vi "Multirecord Acquisition FPGA_20221228a.vi"() -> ()   [LabVIEW 2021]
doc: "Use this VI as a template for the reconfigurable oscilloscope acquisition design. The block diagram is divided into three main loops.\n\nRegister Bus: This loop initializes the registers that are needed to support the configuration of the device. The FIFO bus, on the left, allows all the other design libraries to communicate with one another. This loop is very important to support the proper behavior of the instrument design library components.\n\nAcquisition: Acquires data from the I/O channels and writes the data into the record memory using the <B>Write</B> VI of the Multirecord Acquisition instrument design library. This VI also evaluates the various acquisition triggers and decides whether to acquire each data value in record memory. The host level VI (Fetch Record.vi) can read acquired records from the DRAM. The data is stored in 2 DRAM banks, each with 768 MB of storage.\n\nFetch: The recorded data is retrieved when the <B>Fetch Single Record</B> VI is run from the host VI. The <B>Write to Fetch DMA FIFO</B> VI writes data to the acq.fetch fifo 0 to transmit record data form the FPGA to the record fetch VIs on the host. This DMA FIFO must have a predefined name based on the instance parameter. By default, it is 0 (since the associated terminal on the <B>Create Resources DRAM Write Read</B> VI is unwired), so the connected FIFO is named acq.fetch fifo 0."
uses:
  FPGA Interface Typedefinitions/Trigger Combination Type.ctl
  Host/Clusts/AllWindowsClust.ctl
  Host/Clusts/ChannelWindowClust.ctl
  Controls/Clust/WindowTriggerClust.ctl
  <instrlib>/_niInstr/Data Trigger/v1/Shared/Public/Level Configuration FXP(+-,18,1).ctl
  <instrlib>/_niInstr/Data Trigger/v1/Shared/Public/Level Configuration Trigger When.ctl
  <vilib>/Platform/TimedLoop/XDataNode/timing_clust.ctl
  <vilib>/Platform/TimedLoop/XDataNode/nitl_modes.ctl
  <vilib>/Platform/TimedLoop/XDataNode/wakeup.ctl
  Controls/Clust/All_acquisition_Resources.ctl
  <instrlib>/_niInstr/Multirecord Acquisition/Common/v1/FPGA/niInstr Multirecord Acquisition Common v1 FPGA.lvclass
  C:/Program Files (x86)/National Instruments/LabVIEW 2021/instr.lib/_niInstr/Multirecord Acquisition/Interface/v1/FPGA/niInstr Multirecord Acquisition v1 FPGA.lvclass
  Controls/Clust/Status_Booleans_Clust.ctl
  Controls/Clust/Trig_Config_Clust.ctl
  <instrlib>/_niInstr/FIFO Register Bus/v1/FPGA/niInstr FIFO Register Bus v1 FPGA.lvclass
  C:/Program Files (x86)/National Instruments/LabVIEW 2021/instr.lib/_niInstr/Instruction Framework/v1/FPGA/Interfaces/Instruction Producer/Instruction Producer.lvclass
  <vilib>/rvi/Emulation/niFpgaSctlEmulationGetInTimedLoop.vi
  <vilib>/rvi/Emulation/niFpgaEmulationReportErrorSimple.vi
  <vilib>/rvi/Emulation/niFpgaGetClockAttributes.vi
  <vilib>/rvi/Emulation/niFpgaCriticalErrorInLSC.vi
  <instrlib>/_niInstr/Multirecord Acquisition/Common/v1/FPGA/Private/Create Fetch DMA FIFO Resources U8x32.vi
  <instrlib>/_niInstr/Multirecord Acquisition/Common/v1/FPGA/Private/Create Resources DRAM U384x2 U768 Write Read.vi
  <instrlib>/_niInstr/Multirecord Acquisition/Interface/v1/FPGA/Private/Retrieve Record U16 Wrapper.vi
  <instrlib>/_niInstr/Multirecord Acquisition/Interface/v1/FPGA/Private/Write to Fetch DMA FIFO U16 Wrapper.vi
  <vilib>/rvi/eio/common/nirviEmuTemplateMethod_errors.vi
  <instrlib>/HSAI-RIO/Config/Group A/v1/FPGA/Digital Correction/Validate 8 Channel Data.vi
  <instrlib>/HSAI-RIO/Config/Group A/v1/FPGA/Digital Correction/Digital Correction (8 Ch).vi
  <instrlib>/HSAI-RIO/Config/Group A/v1/FPGA/Digital Correction/FIR Filter (8 Ch).vi
  DSP/SubVIs/Integer decimationx8ch.vi
  <vilib>/Platform/TimedLoop/XDataNode/XDataNode.xnode
  <vilib>/eio/EIONode/EIONode.xnode
  <instrlib>/_niInstr/Instruction Framework/v1/FPGA/Top Level Bus/Register Configuration/Register Configuration.lvclass
  <vilib>/Platform/TimedLoop/XDataNode/XDNodeRunTimeDep.lvlib
  <instrlib>/_niInstr/Multirecord Acquisition/Interface/v1/FPGA/niInstr Multirecord Acquisition v1 FPGA.lvclass
  <instrlib>/_niInstr/Basic Elements/v1/FPGA/niInstr Basic Elements v1 FPGA.lvlib
  <instrlib>/HSAI-RIO/Config/Group A/v1/FPGA/Digital Correction/Digital Correction.lvclass
  <instrlib>/HSAI-RIO/Config/Group A/v1/FPGA/Config Registers/Config Registers.lvclass
  FPGA Interface Typedefinitions/FPGA Interface Typedefinitions.lvlib
  C:/Program Files (x86)/National Instruments/LabVIEW 2021/instr.lib/_niInstr/Multirecord Acquisition/Common/v1/FPGA/niInstr Multirecord Acquisition Common v1 FPGA.lvclass
  Emulation/SubVIs/2 Element Generate Sine Cos Data FXP(+,-,14,1).vi
  <instrlib>/_niInstr/Data Trigger/v1/Shared/niInstr Data Trigger v1 Shared.lvlib
panel:
  in  "channel.enable mask":u16=65535 format="%.0b"
  in  "channel.number of channels":u8=8
  out "overflow 2":bool
  out "TrigCount 2":u32
  out "Trigger Index 2":u16
  out "TrigCfg 1":T1
  out "Trigger Index":u16
  out "TrigCount":u32
  out "TrigCfg 0":T1
  in  "ResetTrig":bool
  in  "UserTrig":T4
  in  "trigger.rearm delay":u16=2
  in  "start trigger":bool=TRUE
  in  "reset":bool
  in  "trigger.combination type":T6
  out "fifo reg bus data 0":u64
  out "fifo reg bus status 0":u32
  in  "fifo reg bus ctrl 0":u32
  out "overflow":bool
  in  "dsp.decimation factor":u16
  out "overload":bool
  # "Register Bus Controls"
  # "FPGA"
  # "DSP"
  # "Trigger"
  # "Unused controls included to make API work"
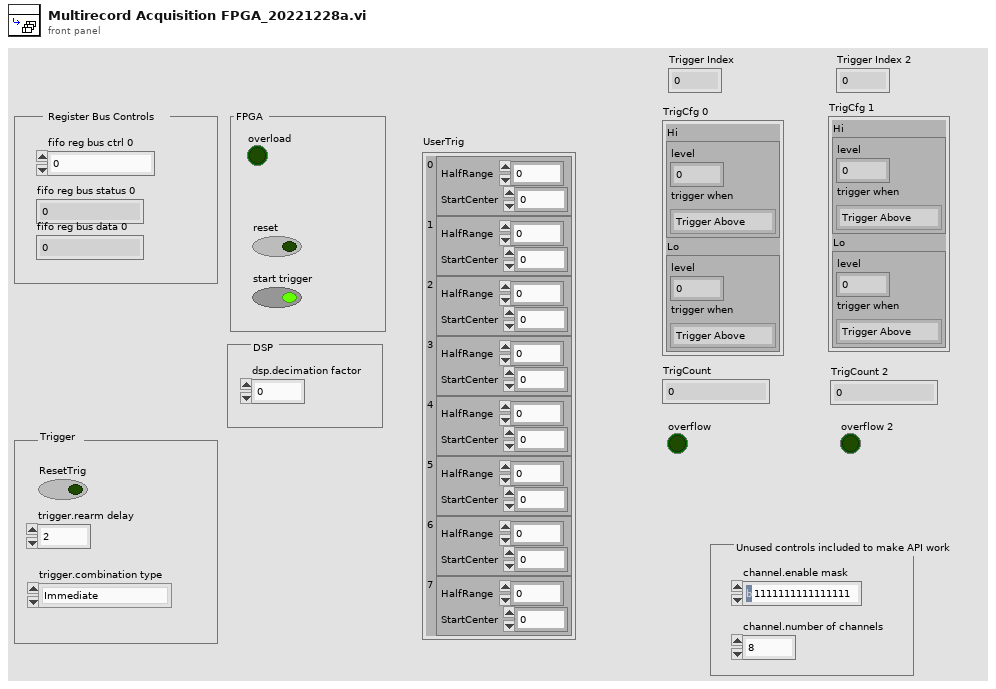
[diagram p1: front panel]
types:
  T1 = typedef "WindowTriggerClust.ctl" = cluster{"Hi":T2, "Lo":T2}
  T2 = typedef "niInstr Data Trigger v1 Shared.lvlib/Level Configuration FXP(+-,18,1).ctl" = cluster{"level":fxp<+/-,18,5>, "trigger when":T3}
  T3 = typedef "niInstr Data Trigger v1 Shared.lvlib/Level Configuration Trigger When.ctl" = enum8{"Trigger Above", "Trigger Below"}
  T4 = typedef "AllWindowsClust.ctl" = cluster{"0":T5, "1":T5, "2":T5, "3":T5, "4":T5, "5":T5, "6":T5, "7":T5}
  T5 = typedef "ChannelWindowClust.ctl" = cluster{"HalfRange":fxp<+/-,18,5>, "StartCenter":fxp<+/-,18,5>}
  T6 = typedef "FPGA Interface Typedefinitions.lvlib/Trigger Combination Type.ctl" = enum16{"Immediate", "A", "B", "OR", "AND", "A THEN B", "B THEN A", "High Resolution"}
  T7 = typedef "All_acquisition_Resources.ctl" = cluster{"FIFO 0":refnum<class "niInstr Multirecord Acquisition Common v1 FPGA.lvclass">, "FIFO 1":refnum<class "niInstr Multirecord Acquisition Common v1 FPGA.lvclass">, "FIFO 2":refnum<class "niInstr Multirecord Acquisition Common v1 FPGA.lvclass">, "FIFO 3":refnum<class "niInstr Multirecord Acquisition Common v1 FPGA.lvclass">, "FIFO 4":refnum<class "niInstr Multirecord Acquisition Common v1 FPGA.lvclass">, "FIFO 5":refnum<class "niInstr Multirecord Acquisition Common v1 FPGA.lvclass">, "FIFO 6":refnum<class "niInstr Multirecord Acquisition Common v1 FPGA.lvclass">, "FIFO 7":refnum<class "niInstr Multirecord Acquisition Common v1 FPGA.lvclass">}
  T8 = cluster{"memory 1":refnum<k21>, "memory 2":refnum<k21>}
  T9 = typedef "XDNodeRunTimeDep.lvlib/timing_clust.ctl" = cluster{"Expected End [f-1]":u64, "Actual End [f-1]":u64, "Finished Late? [f-1]":bool, "Expected End [i-1]":u64, "Actual End [i-1]":u64, "Finished Late? [i-1]":bool, "Expected Start [i]":u64, "Actual Start [i]":u64, "Expected Start [f]":u64, "Actual Start [f]":u64, "Source Name":string, "Structure Name":string, "Period":i64, "Deadline":i64, "Offset":i64, "Start":i64, "Priority":i32, "Timeout":i32, "Mode":T10, "Wakeup Reason":T11, "Error":errorcluster, "Source Type":string, "Secondary Source Type":string, "Global End Time":u64, "Global Start Time":u64, "Frame Duration":u64, "Iteration Duration":u64, "Assigned CPU":i32, "I/O Scan Engine Mode":u32}
  T10 = typedef "XDNodeRunTimeDep.lvlib/nitl_modes.ctl" = enum32{"No Change", "Process missed periods, maintain original phase", "Discard missed periods, maintain original phase", "Process missed periods, ignore original phase", "Discard missed periods, ignore original phase"}
  T11 = typedef "XDNodeRunTimeDep.lvlib/wakeup.ctl" = enum32{"Normal", "Aborted", "Asynchronous wakeup", "Timing source error", "Timed loop error", "Timeout"}
  T12 = typedef "Trig_Config_Clust.ctl" = cluster{"UserTrig":T4, "type":T6, "rearm delay":u16}
  T13 = typedef "Status_Booleans_Clust.ctl" = cluster{"reset out":bool, "ResetTrig":bool, "output valid":bool}
  T14 = cluster{"Channel 0":fxp<+/-,14,1>[], "Channel 1":fxp<+/-,14,1>[], "Channel 2":fxp<+/-,14,1>[], "Channel 3":fxp<+/-,14,1>[], "Channel 4":fxp<+/-,14,1>[], "Channel 5":fxp<+/-,14,1>[], "Channel 6":fxp<+/-,14,1>[], "Channel 7":fxp<+/-,14,1>[]}
  T15 = cluster{"Channel 0":fxp<+/-,18,1>[], "Channel 1":fxp<+/-,18,1>[], "Channel 2":fxp<+/-,18,1>[], "Channel 3":fxp<+/-,18,1>[], "Channel 4":fxp<+/-,18,1>[], "Channel 5":fxp<+/-,18,1>[], "Channel 6":fxp<+/-,18,1>[], "Channel 7":fxp<+/-,18,1>[]}
  T16 = cluster{"channel 0":fxp<+/-,18,1>[], "channel 1":fxp<+/-,18,1>[], "channel 2":fxp<+/-,18,1>[], "channel 3":fxp<+/-,18,1>[], "channel 4":fxp<+/-,18,1>[], "channel 5":fxp<+/-,18,1>[], "channel 6":fxp<+/-,18,1>[], "channel 7":fxp<+/-,18,1>[]}
  T17 = typedef "niInstr Multirecord Acquisition v1 FPGA.lvclass/Retrieve Data Info.ctl" = cluster{"read request size (bits)":u64, "valid data offset (bits)":u16, "valid data size (bits)":u16, "first sample of request":bool, "last sample of request":bool, "Token":T18}
  T18 = typedef "niInstr Types v1 Shared.lvlib/Token.ctl" = cluster{"identifier":u8, "value":u32}
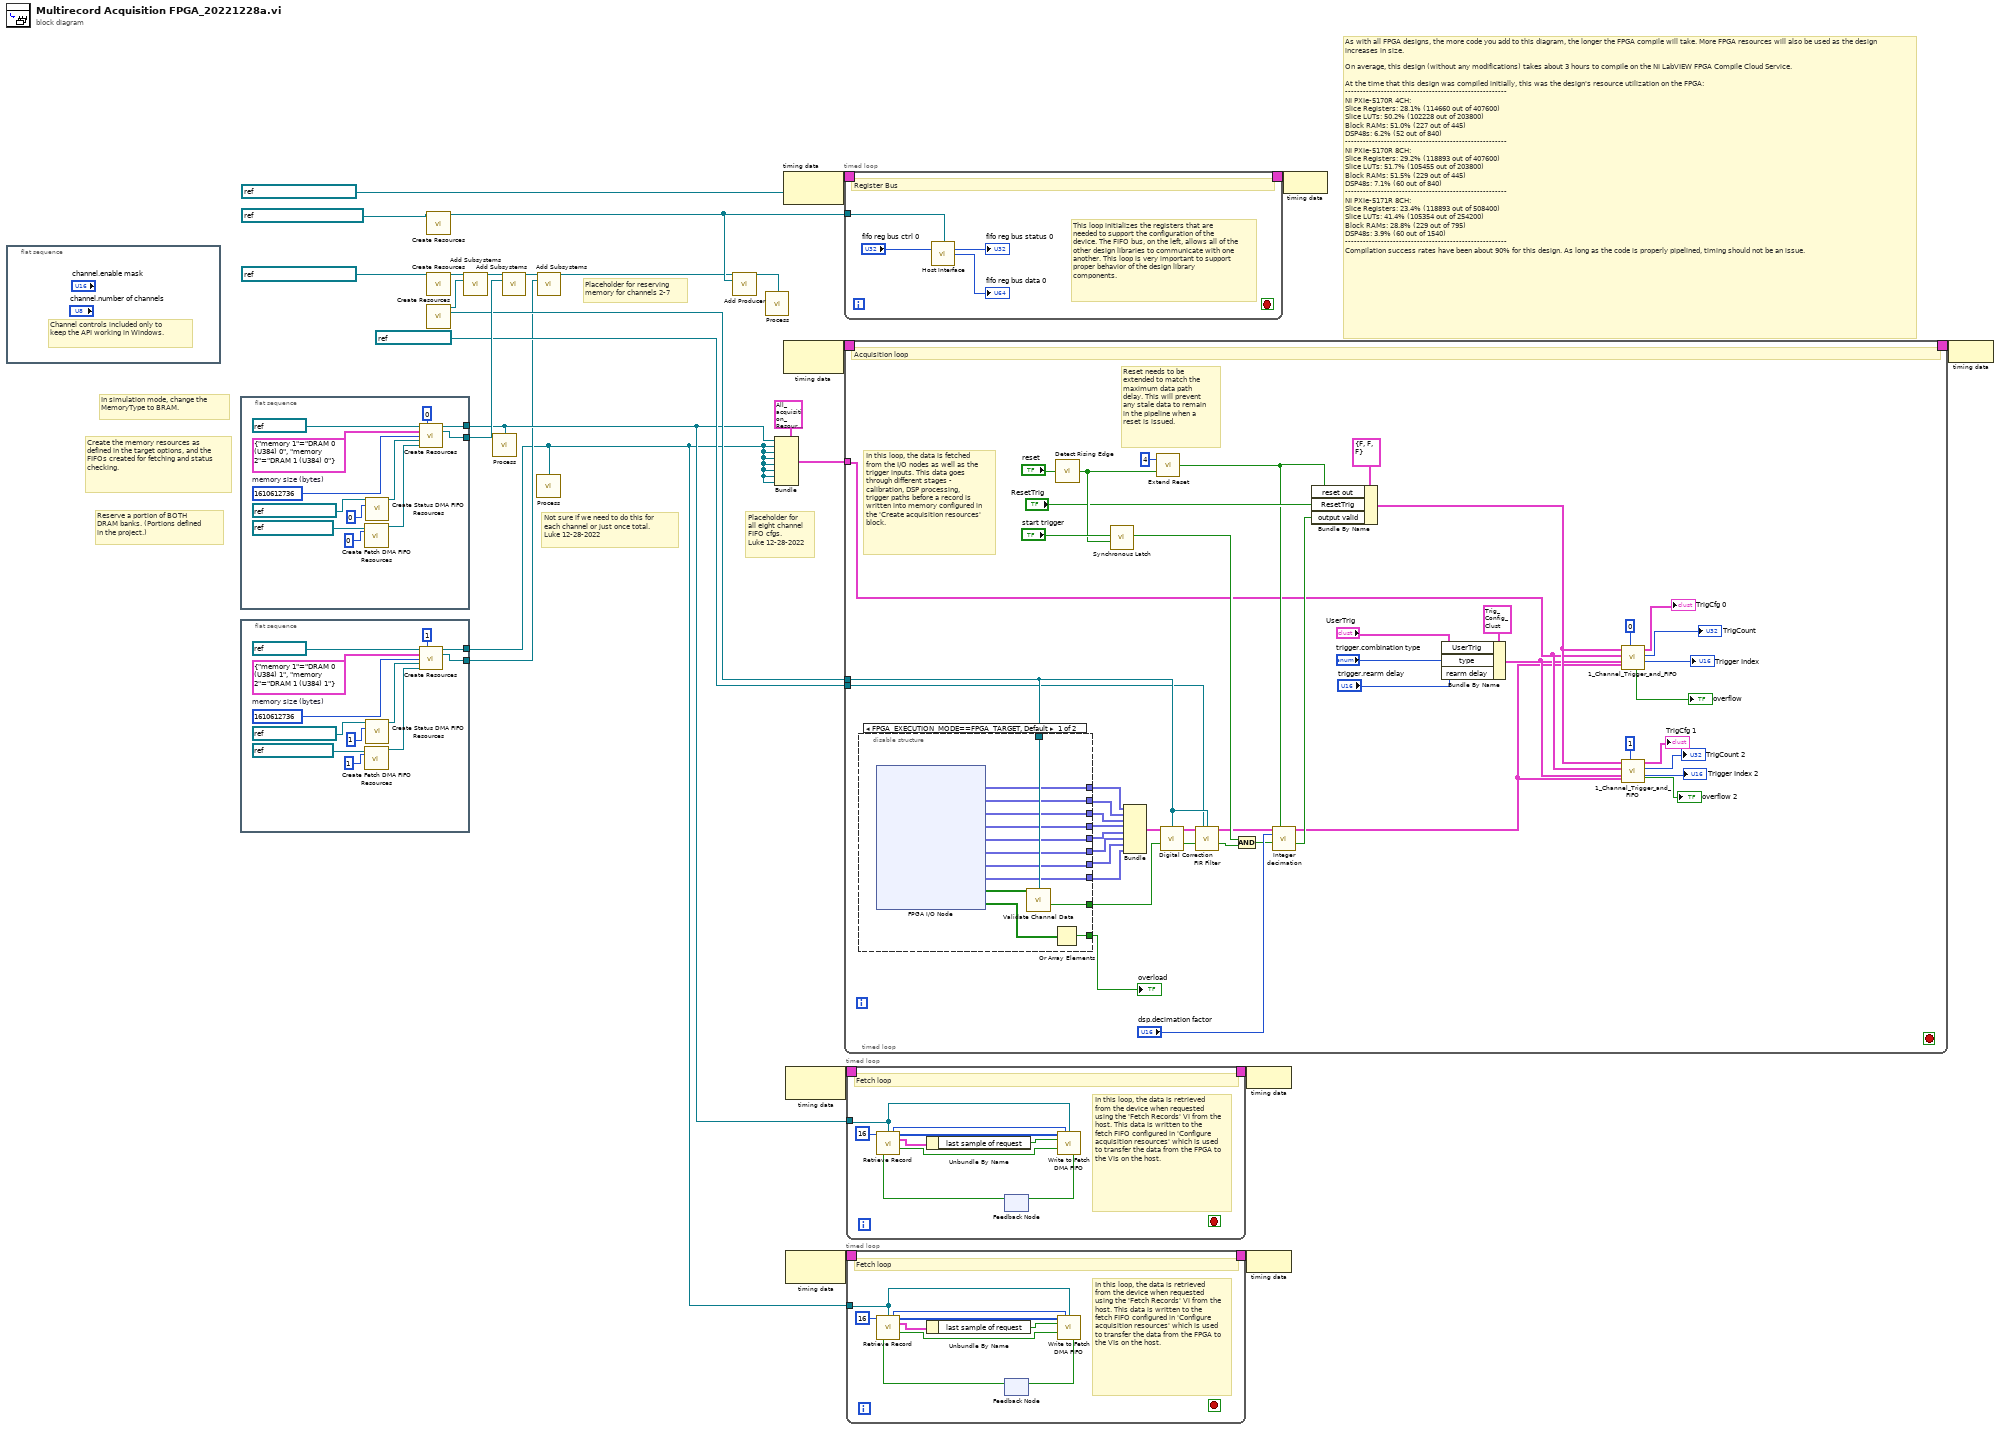
[diagram p0: block diagram]
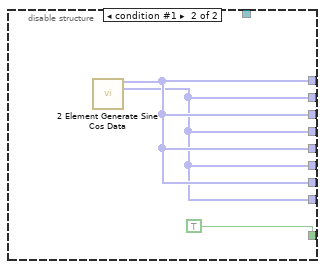
[diagram p2: hidden frame]
diagram:
  # "Not sure if we need to do this for \neach channel or just once total.\nLuke 12-28-2022"
  # "Placeholder for reserving\nmemory for channels 2-7"
  # "Reserve a portion of BOTH\nDRAM banks. (Portions defined\nin the project.)"
  # "Placeholder for\nall eight channel\nFIFO cfgs.\nLuke 12-28-2022"
  # "In simulation mode, change the MemoryType to BRAM."
  # "Create the memory resources as defined in the target options, and the FIFOs created for fetching and status checking."
  # "As with all FPGA designs, the more code you add to this diagram, the longer the FPGA compile will take. More FPGA resources will also be used as the design increases in size.\n\nOn average, this design (without any modifications) takes about 3 hours to compile on the NI LabVIEW FPGA Compile Cloud Service. \n\nAt the time that this design was compiled initially, this was the design's resource utilization on the FPGA:\n------------------------------------------------------\nNI PXIe-5170R 4CH:\nSlice Registers: 28.1% (114660 out of 407600)\nSlice LUTs: 50.2% (102228 out of 203800)\nBlock RAMs: 51.0% (227 out of 445)\nDSP48s: 6.2% (52 out of 840)\n------------------------------------------------------\nNI PXIe-5170R 8CH:\nSlice Registers: 29.2% (118893 out of 407600)\nSlice LUTs: 51.7% (105455 out of 203800)\nBlock RAMs: 51.5% (229 out of 445)\nDSP48s: 7.1% (60 out of 840)\n------------------------------------------------------\nNI PXIe-5171R 8CH:\nSlice Registers: 23.4% (118893 out of 508400)\nSlice LUTs: 41.4% (105354 out of 254200)\nBlock RAMs: 28.8% (229 out of 795)\nDSP48s: 3.9% (60 out of 1540)\n------------------------------------------------------\nCompilation success rates have been about 90% for this design. As long as the code is properly pipelined, timing should not be an issue."
  n1 = flat-sequence {
    frame #0 {
      # "Channel controls included only to keep the API working in Windows."
    }
  }
  n2 = flat-sequence {
    tunnel: [w38] -> w14
    tunnel: [w37] -> w8
    frame #0 {
      w36 = u64 1610612736  # memory size (bytes)
      n3 = call-poly <instrlib>:"Create Fetch DMA FIFO Resources.vi"("fetch dma fifo in"=refnum<k21> "acq.fetch fifo 0", "fifo instance"=u8 0) -> ("fetch dma fifo out"=w34:refnum<class "niInstr Fetch FIFO v1 FPGA.lvclass">)  [unwired: 13 in]
      n4 = call <instrlib>:"Create Status DMA FIFO Resources.vi"("status dma fifo in"=refnum<k21> "acq.status fifo 0" ("status dma fifo"), "fifo instance"=u8 0) -> ("status dma fifo out"=w30:refnum<class "niInstr Status FIFO v1 FPGA.lvclass">)  [unwired: 13 in]
      n5 = call-poly <instrlib>:"Create Resources.vi"("memory clock"=refnum<k21> "160MHz" ("process clock"), "instance"=u8 0, "memory"=T8 {"memory 1"="DRAM 0 (U384) 0", "memory 2"="DRAM 1 (U384) 0"}, "memory size (bytes)"=w36, "status dma fifo resources"=w30, "fetch dma fifo resources"=w34) -> ("acquisition resources"=w37:refnum<class "niInstr Multirecord Acquisition Common v1 FPGA.lvclass">, "acquisition subsystem"=w38:refnum<class "Address Space Collection.lvclass">)  [unwired: 8 in]
    }
  }
  n6 = flat-sequence {
    tunnel: [w50] -> w6
    tunnel: [w49] -> w1
    frame #0 {
      w48 = u64 1610612736  # memory size (bytes)
      n7 = call-poly <instrlib>:"Create Fetch DMA FIFO Resources.vi"("fetch dma fifo in"=refnum<k21> "acq.fetch fifo 1", "fifo instance"=u8 1) -> ("fetch dma fifo out"=w46:refnum<class "niInstr Fetch FIFO v1 FPGA.lvclass">)  [unwired: 13 in]
      n8 = call <instrlib>:"Create Status DMA FIFO Resources.vi"("status dma fifo in"=refnum<k21> "acq.status fifo 1" ("status dma fifo"), "fifo instance"=u8 1) -> ("status dma fifo out"=w42:refnum<class "niInstr Status FIFO v1 FPGA.lvclass">)  [unwired: 13 in]
      n9 = call-poly <instrlib>:"Create Resources.vi"("memory clock"=refnum<k21> "160MHz" ("process clock"), "instance"=u8 1, "memory"=T8 {"memory 1"="DRAM 0 (U384) 1", "memory 2"="DRAM 1 (U384) 1"}, "memory size (bytes)"=w48, "status dma fifo resources"=w42, "fetch dma fifo resources"=w46) -> ("acquisition resources"=w49:refnum<class "niInstr Multirecord Acquisition Common v1 FPGA.lvclass">, "acquisition subsystem"=w50:refnum<class "Address Space Collection.lvclass">)  [unwired: 8 in]
    }
  }
  n10 = call <instrlib>:"Create Resources.vi"("instruction fifo"=refnum<k21> "reg.host instruction fifo 0" ("FIFO")) -> ("fifo register bus"=w13:refnum<class "niInstr FIFO Register Bus v1 FPGA.lvclass">)  [unwired: 14 in]
  n11 = call <instrlib>:"Create Resources.vi"("register clock"=refnum<k21> "40 MHz Onboard Clock" ("Source Name")) -> ("register configuration"=w17:refnum<class "Register Configuration.lvclass">)  [unwired: 14 in]
  n12 = call <instrlib>:"Create Resources.vi"() -> ("config subsystems"=w15:refnum<class "Address Space Collection.lvclass">, "digital correction resources"=w10:refnum<class "Digital Correction.lvclass">)  [unwired: 14 in]
  n13 = call-dynamic "Add Subsystems.vi"("register configuration in"=w17, "subsystems"=w15) -> ("register configuration out"=w16:refnum<class "Register Configuration.lvclass">)  [unwired: 13 in]
  n14 = call-dynamic "Process.vi"("acquisition resources"=w8) -> ()  [unwired: 15 in]
  n15 = call-dynamic "Add Subsystems.vi"("register configuration in"=w16, "subsystems"=w14) -> ("register configuration out"=w5:refnum<class "Register Configuration.lvclass">)  [unwired: 13 in]
  n16 = call-dynamic "Process.vi"("acquisition resources"=w1) -> ()  [unwired: 15 in]
  n17 = call-dynamic "Add Subsystems.vi"("register configuration in"=w5, "subsystems"=w6) -> ("register configuration out"=w4:refnum<class "Register Configuration.lvclass">)  [unwired: 13 in]
  n18 = call-dynamic "Add Producer.vi"("register configuration in"=w4, "instruction producer"=w13) -> ("register configuration out"=w12:refnum<class "Register Configuration.lvclass">)  [unwired: 13 in]
  n19 = call-dynamic "Process.vi"("register configuration"=w12) -> ()  [unwired: 15 in]
  n20 = Bundle(cluster=T7 {"FIFO 0"=refnum, "FIFO 1"=refnum, "FIFO 2"=refnum, "FIFO 3"=refnum, "FIFO 4"=refnum, "FIFO 5"=refnum, "FIFO 6"=refnum, "FIFO 7"=refnum}, "FIFO 0"=w8, "FIFO 1"=w1, "FIFO 2"=w1, "FIFO 3"=w1, "FIFO 4"=w1, "FIFO 5"=w1, "FIFO 6"=w1, "FIFO 7"=w1) -> (w7:T7)
  n21 = node-c288(refnum<k21> "40 MHz Onboard Clock" ("Source Name")) -> (w26:T9)
  n22 = node-c288() -> (w24:T9)  [unwired: 1 in]
  n23 = node-c288() -> (w22:T9)  [unwired: 1 in]
  n24 = node-c288() -> (w3:T9)  [unwired: 1 in]
  n25 = timed-loop {
    timing: w26 -> [_]
    timing-out: [_] -> w25
    tunnel: w13 -> [w54]
    stop <- _ stop-if-true
    # "This loop initializes the registers that are needed to support the configuration of the device. The FIFO bus, on the left, allows all of the other design libraries to communicate with one another. This loop is very important to support proper behavior of the design library components."
    # "Register Bus"
    n26 = call <instrlib>:"Host Interface.vi"("fifo register bus"=w54, "fifo reg bus ctrl 0"="fifo reg bus ctrl 0") -> ("fifo reg bus status 0"=→"fifo reg bus status 0":u32, "fifo reg bus data 0"=→"fifo reg bus data 0":u64)  [unwired: 12 in]
  }
  n27 = timed-loop {
    timing: w24 -> [_]
    timing-out: [_] -> w23
    tunnel: w7 -> [w64]
    tunnel: w10 -> [w97]
    tunnel: refnum<k21> "Data Clock x2" -> [w94]
    stop <- _ stop-if-true
    # "Reset needs to be extended to match the maximum data path delay. This will prevent any stale data to remain in the pipeline when a reset is issued."
    # "In this loop, the data is fetched from the I/O nodes as well as the trigger inputs. This data goes through different stages - calibration, DSP processing, trigger paths before a record is written into memory configured in the 'Create acquisition resources' block."
    # "Acquisition loop"
    n28 = disable-structure shown="FPGA_EXECUTION_MODE==FPGA_TARGET, Default" {
      disable-tunnel: [w113 w118] -> w93
      disable-tunnel: [w112 w117] -> w92
      disable-tunnel: [w111 w118] -> w91
      disable-tunnel: [w110 w117] -> w90
      disable-tunnel: [w109 w118] -> w89
      disable-tunnel: [w108 w117] -> w88
      disable-tunnel: [w107 w118] -> w86
      disable-tunnel: [w106 w117] -> w87
      disable-tunnel: [w103 TRUE ("ADC Data Valid")] -> w84
      disable-tunnel: w97 -> [w114 _]
      disable-tunnel: [w104 _] -> w102
      frame condition #0 (active) {
        # "I/O Nodes"
        n29 = xnode "FPGA I/O Node"() -> ("Channel 0"=w113:fxp<+/-,14,1>[], "Channel 1"=w112:fxp<+/-,14,1>[], "Channel 2"=w111:fxp<+/-,14,1>[], "Channel 3"=w110:fxp<+/-,14,1>[], "Channel 4"=w109:fxp<+/-,14,1>[], "Channel 5"=w108:fxp<+/-,14,1>[], "Channel 6"=w107:fxp<+/-,14,1>[], "Channel 7"=w106:fxp<+/-,14,1>[], "Channel Data Valid"=w115:bool[], "Channel Overload"=w105:bool[])  [unwired: 10 in, 10 out]
        n30 = call-poly <instrlib>:"Validate Channel Data.vi"("channel data valid"=w115, "digital correction resources"=w114) -> ("expected data valid"=w103:bool)  [unwired: 13 in]
        n31 = Or Array Elements(Boolean array=w105) -> (logical OR=w104:bool)
      }
      frame condition #1 {
        n32 = call-poly "2 Element Generate Sine Cos Data.vi"() -> ("sine data"=w118:fxp<+/-,14,1>[], "cosine data"=w117:fxp<+/-,14,1>[])  [unwired: 14 in]
      }
    }
    "overload" <- w102
    n33 = call <instrlib>:"Detect Rising Edge.vi"("signal"="reset") -> ("edge detected"=w96:bool)  [unwired: 14 in]
    n34 = call <instrlib>:"Synchronous Latch.vi"("clear"=w96, "set"="start trigger") -> ("out"=w98:bool)  [unwired: 9 in]
    n35 = Bundle("Channel 0"=w93, "Channel 1"=w92, "Channel 2"=w91, "Channel 3"=w90, "Channel 4"=w89, "Channel 5"=w88, "Channel 6"=w86, "Channel 7"=w87) -> (w85:T14)  [unwired: 1 in]
    n36 = call "Extend Reset.vi"("reset in"=w96, "number of cycles"=u8 4) -> ("reset out"=w75:bool)
    n37 = call-poly <instrlib>:"Digital Correction.vi"("channel data in"=w85, "digital correction resources"=w97, "input valid"=w84) -> ("corrected channel data out"=w82:T15, "output valid"=w81:bool)  [unwired: 11 in]
    n38 = call-poly <instrlib>:"FIR Filter.vi"("data in"=w82, "data clock x2"=w94, "digital correction resources"=w97, "input valid"=w81) -> ("data out"=w79:T15, "output valid"=w80:bool)  [unwired: 9 in, 1 out]
    n39 = And(x=w98, y=w80) -> (x .and. y?=w83:bool)
    n40 = call-poly "Integer decimation.vi"("data in"=w79, "reset"=w75, "decimation factor"="dsp.decimation factor", "input valid"=w83) -> ("data out"=w62:T16, "output valid"=w76:bool)  [unwired: 9 in, 1 out]
    n41 = Bundle By Name(cluster=T13 {"reset out"=FALSE, "ResetTrig"=FALSE, "output valid"=FALSE} ("Status"), "reset out"=w75, "ResetTrig"="ResetTrig", "output valid"=w76) -> (w65:T13)
    n42 = Bundle By Name(cluster=T12 {"UserTrig"={"0"={"HalfRange"=0.0, "StartCenter"=0.0}, "1"={"HalfRange"=0.0, "StartCenter"=0.0}, "2"={"HalfRange"=0.0, "StartCenter"=0.0}, "3"={"HalfRange"=0.0, "StartCenter"=0.0}, "4"={"HalfRange"=0.0, "StartCenter"=0.0}, "5"={"HalfRange"=0.0, "StartCenter"=0.0}, "6"={"HalfRange"=0.0, "StartCenter"=0.0}, "7"={"HalfRange"=0.0, "StartCenter"=0.0}}, "type"=enum."Immediate", "rearm delay"=0} ("output cluster"), "UserTrig"="UserTrig", "type"="trigger.combination type", "rearm delay"="trigger.rearm delay") -> (w63:T12)
    n43 = call "1_Channel_Trigger_and_FIFO.vi"("data in"=w62, "Channel"=i8 0, "Trig Cfg"=w63, "FIFO Cfg"=w64, "Status"=w65) -> ("Trigger Index"=→"Trigger Index":u16, "TrigCount"=→"TrigCount":u32, "TrigCfg"=→"TrigCfg 0":T1, "overflow"=→"overflow":bool)  [unwired: 3 in]
    n44 = call "1_Channel_Trigger_and_FIFO.vi"("data in"=w62, "Channel"=i8 1, "Trig Cfg"=w63, "FIFO Cfg"=w64, "Status"=w65) -> ("Trigger Index"=→"Trigger Index 2":u16, "TrigCount"=→"TrigCount 2":u32, "TrigCfg"=→"TrigCfg 1":T1, "overflow"=→"overflow 2":bool)  [unwired: 3 in]
  }
  n45 = timed-loop {
    timing: w22 -> [_]
    timing-out: [_] -> w21
    tunnel: w8 -> [w129]
    stop <- _ stop-if-true
    # "In this loop, the data is retrieved from the device when requested using the 'Fetch Records' VI from the host. This data is written to the fetch FIFO configured in 'Configure acquisition resources' which is used to transfer the data from the FPGA to the VIs on the host."
    # "Fetch loop"
    n46 = feedback #1() -> (w127:bool)  [unwired: 1 in]
    n47 = call-poly <instrlib>:"Retrieve Record.vi"("output array size"=u16 16, "acquisition resources"=w129, "ready for output"=w127) -> ("channels"=w122:u8, "data"=w125:u16[], "retrieve data info"=w124:T17, "output valid"=w126:bool)  [unwired: 9 in]
    n48 = Unbundle By Name(w124) -> ("last sample of request"=w123:bool)
    n49 = call-poly <instrlib>:"Write to Fetch DMA FIFO.vi"("data"=w125, "channels"=w122, "acquisition resources"=w129, "last sample of request"=w123, "input valid"=w126) -> ("ready for input"=w128:bool)  [unwired: 10 in]
    n50 = feedback-in #1(w128) -> ()
  }
  n51 = timed-loop {
    timing: w3 -> [_]
    timing-out: [_] -> w2
    tunnel: w1 -> [w140]
    stop <- _ stop-if-true
    # "In this loop, the data is retrieved from the device when requested using the 'Fetch Records' VI from the host. This data is written to the fetch FIFO configured in 'Configure acquisition resources' which is used to transfer the data from the FPGA to the VIs on the host."
    # "Fetch loop"
    n52 = feedback #2() -> (w138:bool)  [unwired: 1 in]
    n53 = call-poly <instrlib>:"Retrieve Record.vi"("output array size"=u16 16, "acquisition resources"=w140, "ready for output"=w138) -> ("channels"=w133:u8, "data"=w136:u16[], "retrieve data info"=w135:T17, "output valid"=w137:bool)  [unwired: 9 in]
    n54 = Unbundle By Name(w135) -> ("last sample of request"=w134:bool)
    n55 = call-poly <instrlib>:"Write to Fetch DMA FIFO.vi"("data"=w136, "channels"=w133, "acquisition resources"=w140, "last sample of request"=w134, "input valid"=w137) -> ("ready for input"=w139:bool)  [unwired: 10 in]
    n56 = feedback-in #2(w139) -> ()
  }
  n57 = node-c288(w21) -> ()
  n58 = node-c288(w2) -> ()
  n59 = node-c288(w25) -> ()
  n60 = node-c288(w23) -> ()
